vi "Calculations---.vi"(10 "angle":dbl, 11 "distance":dbl) -> (2 "Knight":T1, 3 "Queen":cluster{"Distance":dbl, "Angle":dbl})   [LabVIEW 2015]
panel:
  in  "Knight 2":T1
  in  "queen 2":cluster{"Distance":dbl, "Angle":dbl}
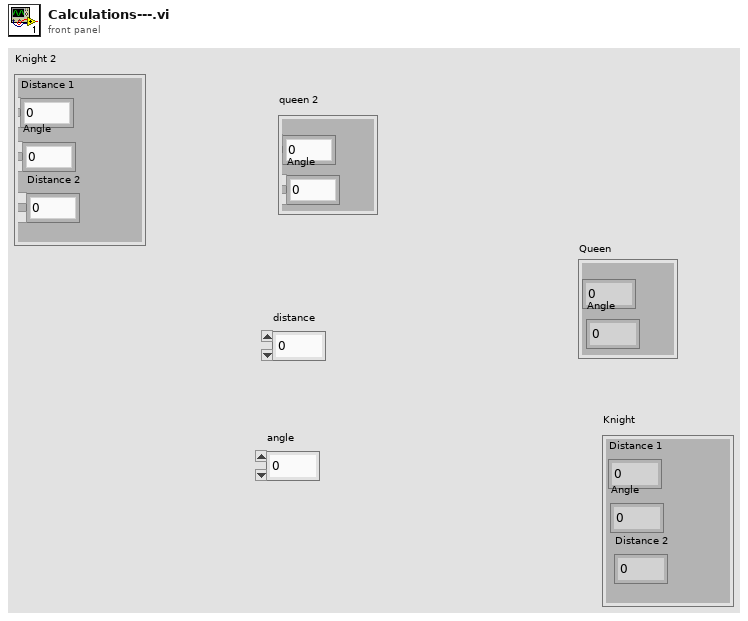
[diagram p1: front panel]
types:
  T1 = cluster{"Distance 1":dbl, "Angle":dbl, "Distance 2":dbl}
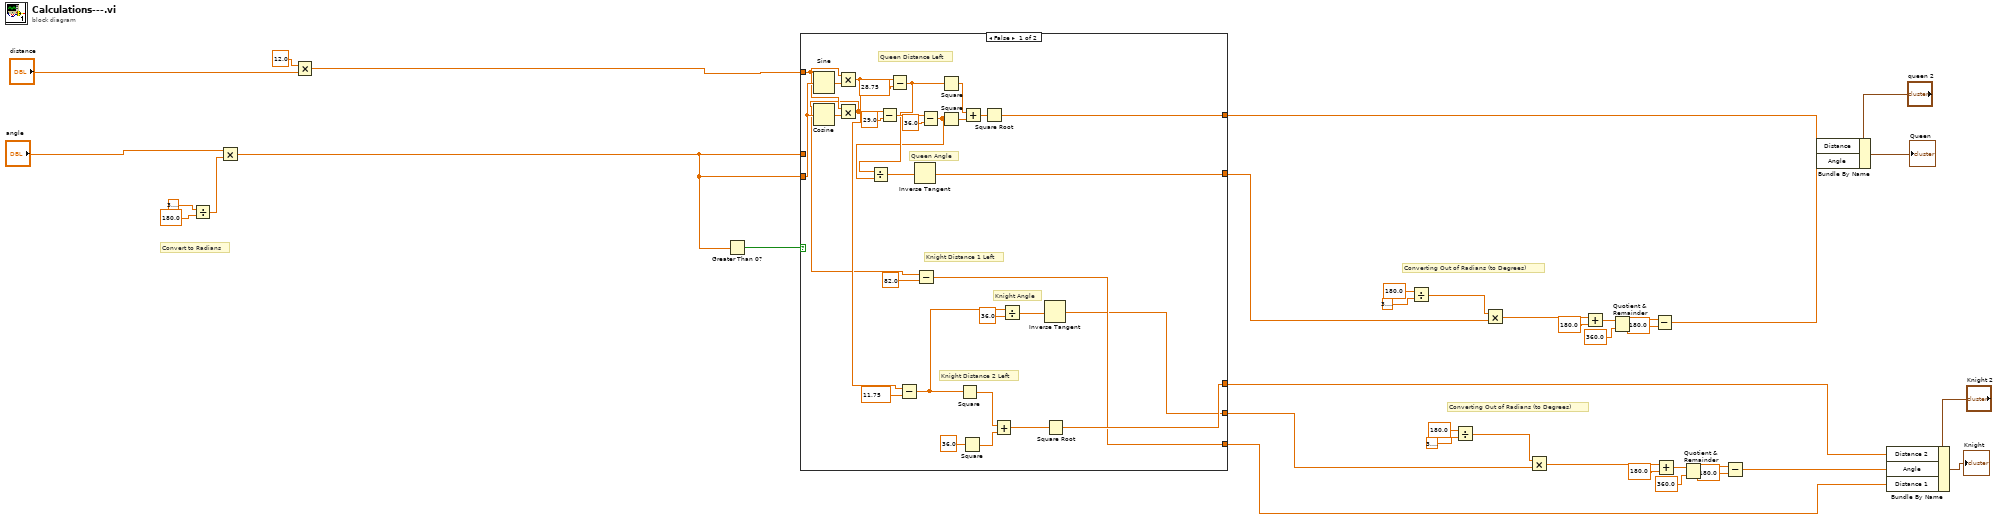
[diagram p0: block diagram]
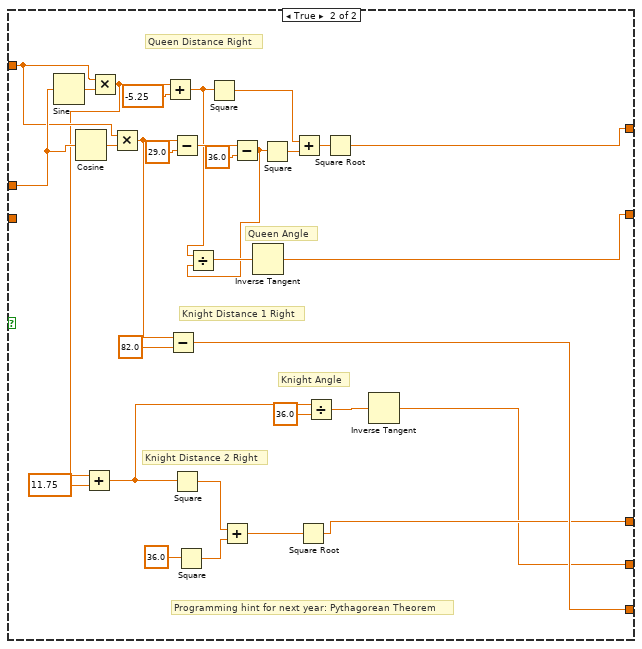
[diagram p2: hidden frame]
diagram:
  # "Converting Out of Radians (to Degrees)"
  # "Converting Out of Radians (to Degrees)"
  # "Convert to Radians"
  n1 = Divide(x=3.141592653589793, y=180.0) -> (x/y=w27:dbl)
  n2 = Multiply(x="angle", y=w27) -> (x*y=w30:dbl)
  n3 = Multiply(x=12.0, y="distance") -> (x*y=w17:dbl)
  n4 = Greater Than 0?(x=w30) -> (x > 0?=w1:bool)
  n5 = case shown="False" w1 {
    tunnel: w30 -> [w54 _]
    tunnel: w17 -> [w53 w88]
    tunnel: [w59 w87] -> w32
    tunnel: [w55 w83] -> w23
    tunnel: w30 -> [_ w90]
    tunnel: [w44 w80] -> w33
    tunnel: [w48 w75] -> w34
    tunnel: [w39 w70] -> w19
    frame False {
      # "Knight Angle"
      # "Knight Distance 1 Left"
      # "Knight Distance 2 Left"
      # "Queen Angle"
      # "Queen Distance Left"
      n6 = Sine(x=w54) -> (sin(x)=w67:dbl)
      n7 = Cosine(x=w54) -> (cos(x)=w62:dbl)
      n8 = Multiply(x=w53, y=w67) -> (x*y=w47:dbl)
      n9 = Multiply(x=w53, y=w62) -> (x*y=w45:dbl)
      n10 = Subtract(x=w45, y=29.0) -> (x-y=w65:dbl)
      n11 = Subtract(x=w47, y=28.75 ("x")) -> (x-y=w58:dbl)
      n12 = Subtract(x=w47, y=11.75) -> (x-y=w42:dbl)
      n13 = Subtract(x=w45, y=82.0) -> (x-y=w44:dbl)
      n14 = Subtract(x=w65, y=36.0) -> (x-y=w57:dbl)
      n15 = Divide(x=w58, y=w57) -> (x/y=w56:dbl)
      n16 = Inverse Tangent(1:w56) -> (0:w55:dbl)
      n17 = Square(x=w58) -> (x^2=w66:dbl)
      n18 = Square(x=w57) -> (x^2=w61:dbl)
      n19 = Square(x=w42) -> (x^2=w52:dbl)
      n20 = Square(x=36.0) -> (x^2=w51:dbl)
      n21 = Add(x=w66, y=w61) -> (x+y=w60:dbl)
      n22 = Square Root(x=w60) -> (sqrt(x)=w59:dbl)
      n23 = Add(x=w52, y=w51) -> (x+y=w43:dbl)
      n24 = Divide(x=w42, y=36.0) -> (x/y=w40:dbl)
      n25 = Inverse Tangent(1:w40) -> (0:w39:dbl)
      n26 = Square Root(x=w43) -> (sqrt(x)=w48:dbl)
    }
    frame True {
      # "Knight Angle"
      # "Programming hint for next year: Pythagorean Theorem"
      # "Knight Distance 2 Right"
      # "Knight Distance 1 Right"
      # "Queen Distance Right"
      # "Queen Angle"
      n27 = Sine(x=w90) -> (sin(x)=w97:dbl)
      n28 = Cosine(x=w90) -> (cos(x)=w93:dbl)
      n29 = Multiply(x=w88, y=w97) -> (x*y=w74:dbl)
      n30 = Add(x=w74, y=11.75) -> (x+y=w69:dbl)
      n31 = Multiply(x=w88, y=w93) -> (x*y=w82:dbl)
      n32 = Add(x=w74, y=-5.25 ("x")) -> (x+y=w85:dbl)
      n33 = Subtract(x=w82, y=82.0) -> (x-y=w80:dbl)
      n34 = Subtract(x=w82, y=29.0) -> (x-y=w96:dbl)
      n35 = Square(x=w69) -> (x^2=w79:dbl)
      n36 = Square(x=36.0) -> (x^2=w78:dbl)
      n37 = Square(x=w85) -> (x^2=w89:dbl)
      n38 = Add(x=w79, y=w78) -> (x+y=w77:dbl)
      n39 = Subtract(x=w96, y=36.0) -> (x-y=w84:dbl)
      n40 = Divide(x=w85, y=w84) -> (x/y=w86:dbl)
      n41 = Inverse Tangent(1:w86) -> (0:w83:dbl)
      n42 = Square(x=w84) -> (x^2=w92:dbl)
      n43 = Add(x=w89, y=w92) -> (x+y=w91:dbl)
      n44 = Square Root(x=w77) -> (sqrt(x)=w75:dbl)
      n45 = Divide(x=w69, y=36.0) -> (x/y=w71:dbl)
      n46 = Square Root(x=w91) -> (sqrt(x)=w87:dbl)
      n47 = Inverse Tangent(1:w71) -> (0:w70:dbl)
    }
  }
  n48 = Divide(x=180.0, y=3.141592653589793) -> (x/y=w24:dbl)
  n49 = Divide(x=180.0, y=3.141592653589793) -> (x/y=w20:dbl)
  n50 = Multiply(x=w24, y=w23) -> (x*y=w9:dbl)
  n51 = Multiply(x=w20, y=w19) -> (x*y=w3:dbl)
  n52 = Add(x=w9, y=180.0) -> (x+y=w14:dbl)
  n53 = Quotient & Remainder(x=w14, y=360.0) -> (x-y*floor(x/y)=w12:dbl)  [unwired: 1 out]
  n54 = Subtract(x=w12, y=180.0) -> (x-y=w10:dbl)
  n55 = Add(x=w3, y=180.0) -> (x+y=w7:dbl)
  n56 = Quotient & Remainder(x=w7, y=360.0) -> (x-y*floor(x/y)=w5:dbl)  [unwired: 1 out]
  n57 = Subtract(x=w5, y=180.0) -> (x-y=w2:dbl)
  n58 = Bundle By Name(cluster="queen 2", "Distance"=w32, "Angle"=w10) -> (→"Queen":cluster{"Distance":dbl, "Angle":dbl})
  n59 = Bundle By Name(cluster="Knight 2", "Distance 2"=w34, "Angle"=w2, "Distance 1"=w33) -> (→"Knight":T1)
